vi "XML Script - Append Terminal Name (Case Selector).vi"(1 "case":string) -> (0 "case.Case Selector":string)   [LabVIEW 2020]
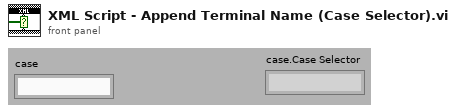
[diagram p1: front panel]
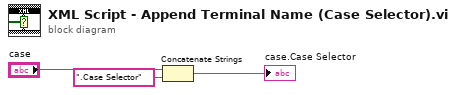
[diagram p0: block diagram]
diagram:
  n1 = Concatenate Strings("case", ".Case Selector" ("string")) -> (→"case.Case Selector":string)
